vi "TuneFeedForward.vi"() -> ()   [LabVIEW 2019]
uses:
  <vilib>/Utility/file.llb/Write Delimited Spreadsheet (DBL).vi
panel:
  out "Good Array":dbl[][](array[numeric])
  out "Array 3":dbl[](array[numeric])
  in  "Next 2.0":bool
  in  "Velocity":dbl
  in  "Power":dbl
  in  "Calibrate":bool
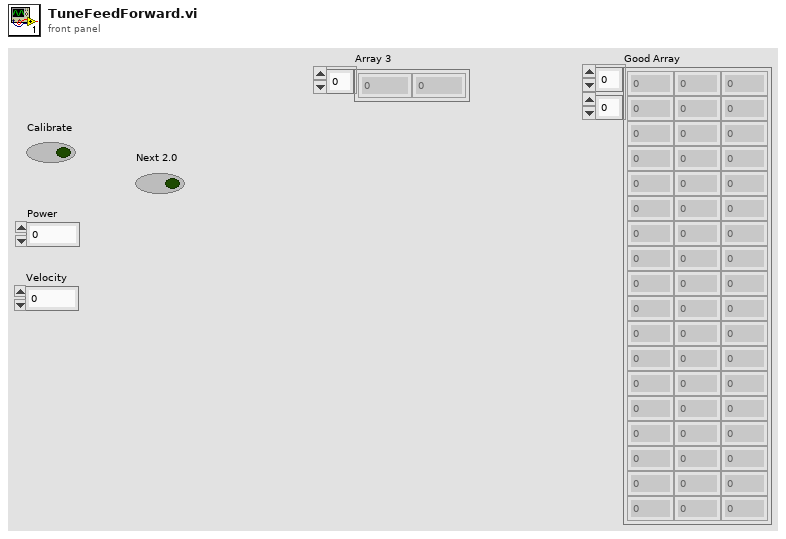
[diagram p1: front panel]
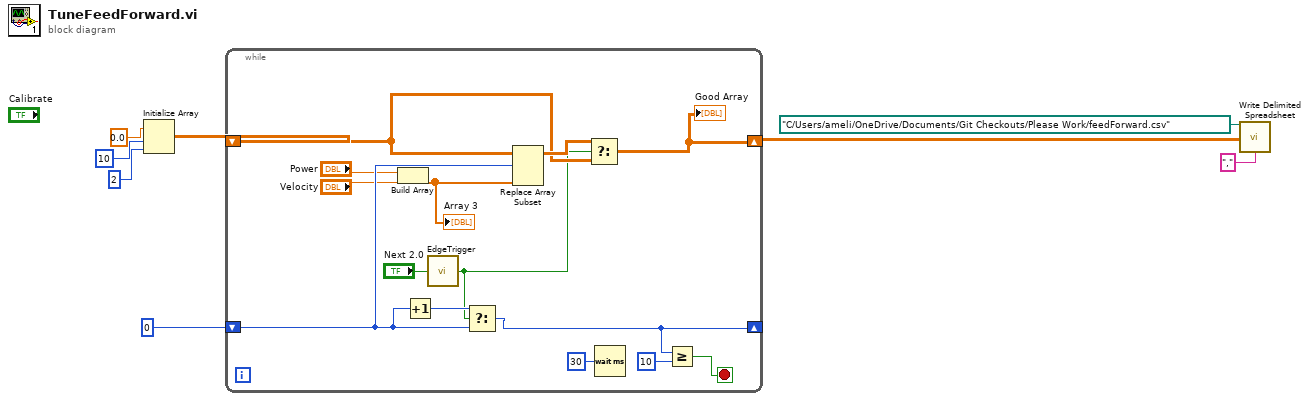
[diagram p0: block diagram]
diagram:
  n1 = Initialize Array(0.0 ("element"), 10 ("dimension size"), 2 ("dimension size")) -> (w6:dbl[][])
  n2 = while {
    shift-right: [w11] -> w3
    shift-left: w6 -> [w21]
    shift-right: [w16] -> _
    shift-left: 0 -> [w13]
    stop <- w14 stop-if-true
    n3 = Build Array("Power", "Velocity") -> (w17:dbl[])
    "Array 3" <- w17
    n4 = Increment(x=w13) -> (x+1=w20:i32)
    n5 = call "EdgeTrigger.vi"("Input Signal"="Next 2.0") -> ("All Edge Trigger"=w12:bool)  [unwired: 2 out]
    n6 = Select(t=w20, s=w12, f=w13) -> (s? t:f=w16:i32)
    n7 = Replace Array Subset(array=w21, new element=w17, index (row)=w13) -> (w22:dbl[][])  [unwired: 1 in]
    n8 = Select(t=w22, s=w12, f=w21) -> (s? t:f=w11:dbl[][])
    "Good Array" <- w11
    n9 = Wait (ms)(milliseconds to wait=u32 30) -> ()  [unwired: 1 out]
    n10 = Greater Or Equal?(x=w16, y=10) -> (x >= y?=w14:bool)
  }
  n11 = call-poly <vilib>:"Write Delimited Spreadsheet.vi"("file path (dialog if empty)"=path "C:/Users/ameli/OneDrive/Documents/Git Checkouts/Please Work/feedForward.csv", "2D data"=w3, "delimiter (\\t)"="," ("delimiter (\\t)")) -> ()  [unwired: 11 in, 2 out]
